vi "StrainMaxMin.vi"(8 "error in (no error)":errorcluster, 9 "Ignore Cal?":bool, 11 "Strain in":refnum<class "Strain.lvclass">) -> (0 "error out":errorcluster, 1 "Min":dbl, 2 "Precision (Max)":i32, 3 "Max":dbl, 4 "Precision (Min)":i32, 5 "Actual Min":dbl, 7 "Actual Max":dbl)   [LabVIEW 2018, in "Measurement Channels.lvlib" / "Strain.lvclass"]
uses:
  Strain.lvclass
  C:/Users/Jeff Tipps/Documents/DAQMan/source/Classes/Measurements/Class Channel/Channel.lvclass
  Strain.lvclass/Strain.ctl
  Class Channel/Read Device.vi
  <vilib>/Utility/TradDaqScaling.llb/Convert Strain Gauge Reading (scaler).vi
panel:
  out "Bridge Configuration\n(3:Half Bridge II)":u16(ring)=6 items=["Qtr Bridge I", "Qtr Bridge II", "Half Bridge I", "Half Bridge II", "Full Bridge I", "Full Bridge II", "Full Bridge III"]
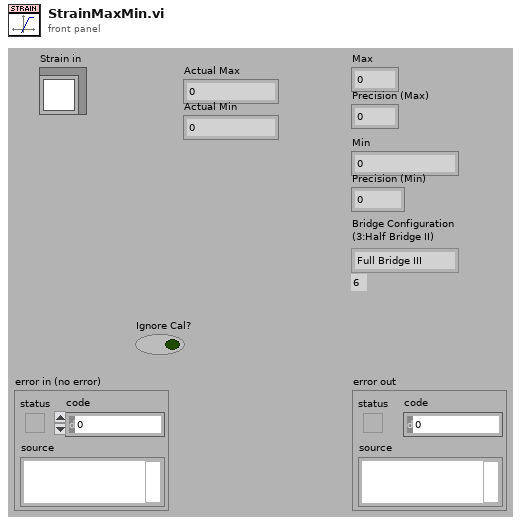
[diagram p1: front panel]
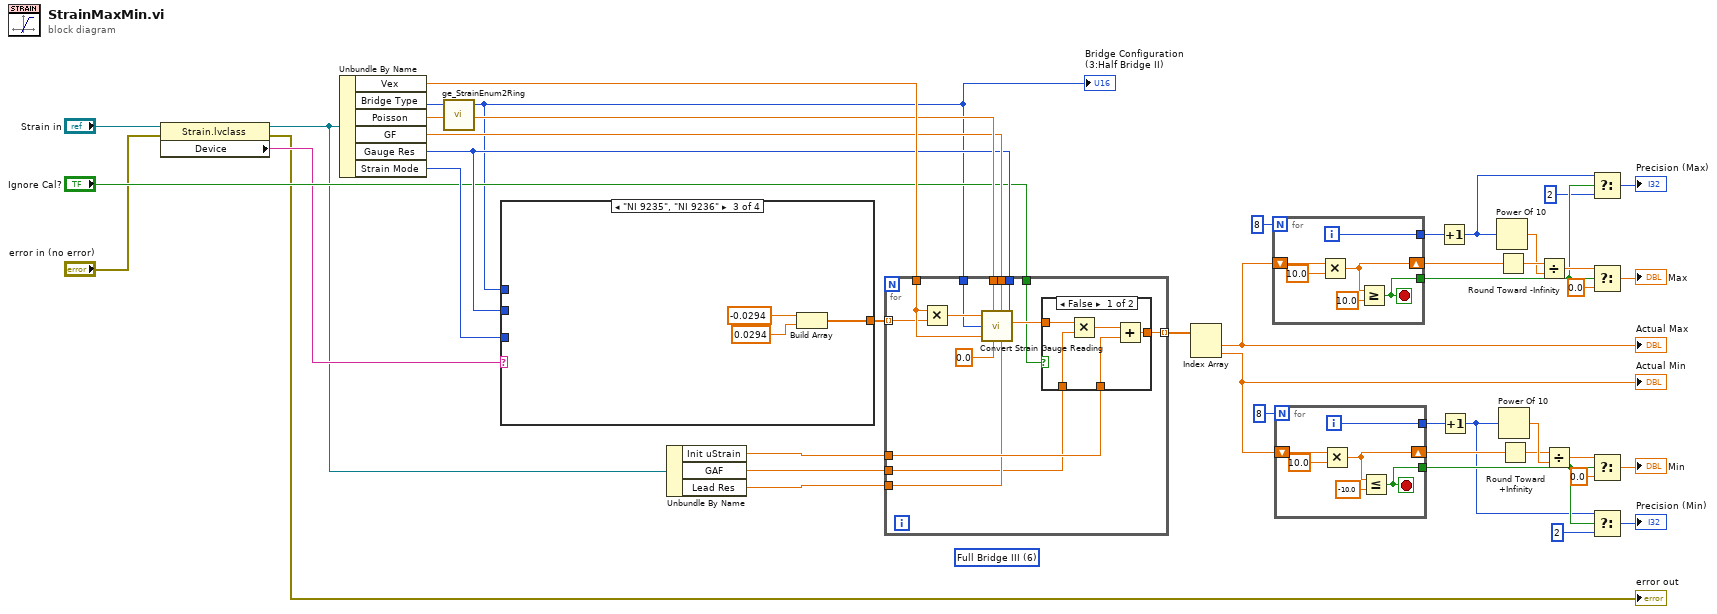
[diagram p0: block diagram]
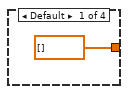
[diagram p3: hidden frame]
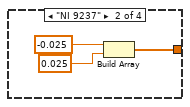
[diagram p4: hidden frame]
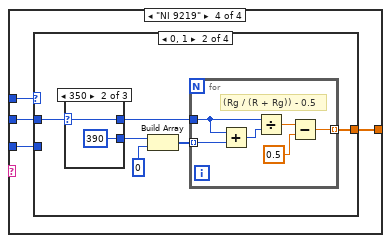
[diagram p5: hidden frame]
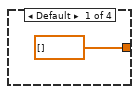
[diagram p6: hidden frame]
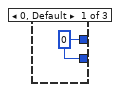
[diagram p7: hidden frame]
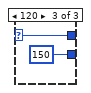
[diagram p8: hidden frame]
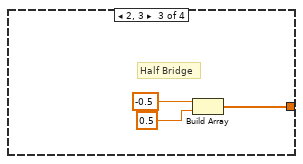
[diagram p9: hidden frame]
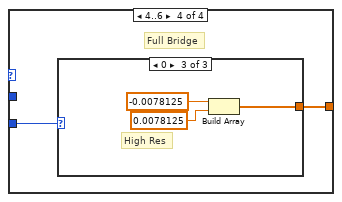
[diagram p10: hidden frame]
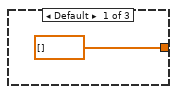
[diagram p11: hidden frame]
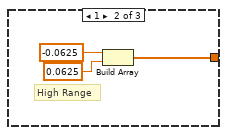
[diagram p12: hidden frame]
diagram:
  (unwired) u16 6 items=["Qtr Bridge I", "Qtr Bridge II", "Half Bridge I", "Half Bridge II", "Full Bridge I", "Full Bridge II", "Full Bridge III"] ("Bridge Configuration\n(3:Half Bridge II)")
  n1 = property class="Strain.lvclass"(reference="Strain in", error in="error in (no error)") -> (reference out=w1:refnum<class "Strain.lvclass">, error out=→"error out":errorcluster, "Device"=w4:string)
  n2 = Unbundle By Name(w1) -> ("Vex"=w44:dbl, "Bridge Type"=w43:u16, "Poisson"=w42:dbl, "GF"=w41:dbl, "Gauge Res"=w35:i32, "Strain Mode"=w36:u16)
  n3 = call "ge_StrainEnum2Ring.vi"("Bridge Type"=w43) -> ("Bridge Config Ring"=w21:u16)  [unwired: 4 in]
  "Bridge Configuration\n(3:Half Bridge II)" <- w21
  n4 = case shown="\"NI 9235\", \"NI 9236\"" w4 {
    tunnel: [dbl[] [] w48 w51 w55] -> w40
    tunnel: w21 -> [_ _ _ w54]
    tunnel: w36 -> [_ _ _ w53]
    tunnel: w35 -> [_ _ _ w52]
    frame Default {
    }
    frame "NI 9237" {
      n5 = Build Array(-0.025, 0.025) -> (w48:dbl[])
    }
    frame "NI 9235", "NI 9236" {
      n6 = Build Array(-0.0294, 0.0294) -> (w51:dbl[])
    }
    frame "NI 9219" {
      n7 = case shown="0, 1" w54 {
        tunnel: [dbl[] [] w60 w76 w78] -> w55
        tunnel: w53 -> [_ _ _ w77]
        tunnel: w52 -> [_ w62 _ _]
        frame Default {
        }
        frame 0, 1 {
          n8 = case shown="350" w62 {
            selector: w62 -> [_ w71 w72]
            tunnel: [w69 390 ("y") 150 ("y")] -> w59
            tunnel: [w69 w71 w72] -> w57
            frame 0, Default {
              w69 = 0 ("Gauge Res")
            }
            frame 350 {
            }
            frame 120 {
            }
          }
          n9 = Build Array(w59, 0 ("Gauge Res")) -> (w61:i32[])
          n10 = for {
            tunnel: [w65] -> w60 mode=indexing
            tunnel: w57 -> [w64]
            tunnel: w61 -> [w63] mode=indexing
            # "(Rg / (R + Rg)) - 0.5"
            n11 = Add(x=w64, y=w63) -> (x+y=w66:i32)
            n12 = Divide(x=w64, y=w66) -> (x/y=w67:dbl)
            n13 = Subtract(x=w67, y=0.5) -> (x-y=w65:dbl)
          }
        }
        frame 2, 3 {
          # "Half Bridge"
          n14 = Build Array(-0.5, 0.5) -> (w76:dbl[])
        }
        frame 4..6 {
          # "Full Bridge"
          n15 = case shown="0" w77 {
            tunnel: [dbl[] [] w82 w85] -> w78
            frame Default {
            }
            frame 1 {
              # "High Range"
              n16 = Build Array(-0.0625, 0.0625) -> (w82:dbl[])
            }
            frame 0 {
              # "High Res"
              n17 = Build Array(-0.0078125, 0.0078125) -> (w85:dbl[])
            }
          }
        }
      }
    }
  }
  n18 = Unbundle By Name(w1) -> ("Init uStrain"=w6:dbl, "GAF"=w37:dbl, "Lead Res"=w38:dbl)
  n19 = for {
    tunnel: w44 -> [w93]
    tunnel: w42 -> [w98]
    tunnel: w41 -> [w97]
    tunnel: w35 -> [w96]
    tunnel: w6 -> [w95]
    tunnel: w21 -> [w87]
    tunnel: w40 -> [w92] mode=indexing
    tunnel: [w91] -> w39 mode=indexing
    tunnel: w38 -> [w90]
    tunnel: w37 -> [w88]
    tunnel: "Ignore Cal?" -> [w86]
    n20 = Multiply(x=w93, y=w92) -> (x*y=w99:dbl)
    n21 = call-poly <vilib>:"Convert Strain Gauge Reading.vi"("Vsg (0.0)"=w99, "v (0.0)"=w98, "Bridge Configuration\n(3:Half Bridge II)"=w87, "Vex (3.33)"=w93, "Vinit (0.0)"=sgl 0.0, "GF (2.0)"=w97, "Rg (120)"=w96, "Rl (0.0)"=w90) -> ("Strain"=w89:sgl)  [unwired: 2 in]
    n22 = case shown="False" w86 {
      tunnel: w95 -> [w104 _]
      tunnel: [w103 w105] -> w91
      tunnel: w89 -> [w102 w105]
      tunnel: w88 -> [w101 _]
      frame False {
        n23 = Multiply(x=w102, y=w101) -> (x*y=w100:dbl)
        n24 = Add(x=w100, y=w104) -> (x+y=w103:dbl)
      }
      frame True {
      }
    }
  }
  n25 = Index Array(array=w39) -> (element #1=w26:dbl, element #2=w25:dbl)  [unwired: 2 in]
  "Actual Max" <- w26
  "Actual Min" <- w25
  n26 = for {
    N: 8 -> [_]
    tunnel: [w107] -> w23
    shift-right: [w108] -> w33
    shift-left: w26 -> [w111]
    tunnel: [w106] -> w17
    i -> [w107]
    stop <- w106 stop-if-true
    n27 = Multiply(x=w111, y=10.0) -> (x*y=w108:dbl)
    n28 = Greater Or Equal?(x=w108, y=10.0) -> (x >= y?=w106:bool)
  }
  n29 = for {
    N: 8 -> [_]
    tunnel: [w113] -> w24
    shift-right: [w114] -> w28
    shift-left: w25 -> [w117]
    tunnel: [w112] -> w10
    i -> [w113]
    stop <- w112 stop-if-true
    n30 = Multiply(x=w117, y=10.0) -> (x*y=w114:dbl)
    n31 = Less Or Equal?(x=w114, y=-10.0) -> (x <= y?=w112:bool)
  }
  n32 = Increment(x=w23) -> (x+1=w16:i32)
  n33 = Increment(x=w24) -> (x+1=w9:i32)
  n34 = Power Of 10(x=w16) -> (10^x=w31:dbl)
  n35 = Round Toward -Infinity(1:w33) -> (0:w32:dbl)
  n36 = Power Of 10(x=w9) -> (10^x=w30:dbl)
  n37 = Round Toward +Infinity(x=w28) -> (ceil(x): smallest int >= x=w29:dbl)
  n38 = Divide(x=w32, y=w31) -> (x/y=w20:dbl)
  n39 = Divide(x=w29, y=w30) -> (x/y=w12:dbl)
  n40 = Select(t=w16, s=w17, f=2) -> (s? t:f=→"Precision (Max)":i32)
  n41 = Select(t=w20, s=w17, f=0.0) -> (s? t:f=→"Max":dbl)
  n42 = Select(t=w12, s=w10, f=0.0) -> (s? t:f=→"Min":dbl)
  n43 = Select(t=w9, s=w10, f=2) -> (s? t:f=→"Precision (Min)":i32)
